vi "workbook.created_at.vi"(8 "error in":errorcluster, 11 "Workbook in":refnum<class "Workbook.lvclass">) -> (0 "error out":errorcluster, 3 "Workbook out":refnum<class "Workbook.lvclass">)   [LabVIEW 2020, in "Workbook.lvclass"]
doc: "Returns the workbook's creation time."
uses:
  Workbook.lvclass
  client.lvlib
panel:
  out "out_millis out":dbl
  in  "out_millis":dbl
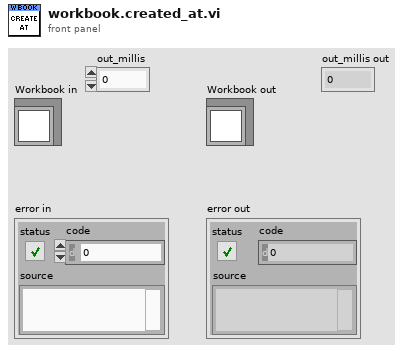
[diagram p1: front panel]
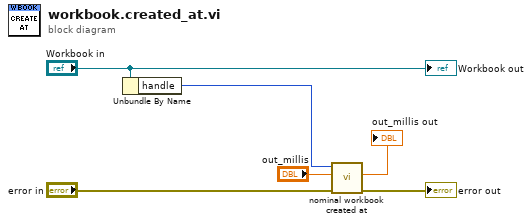
[diagram p0: block diagram]
diagram:
  n1 = Unbundle By Name("Workbook in") -> ("handle"=w4:i32)
  n2 = call "nominal workbook created at.vi"("error in (no error)"="error in", "out_millis"="out_millis", "workbook"=w4) -> ("error out"=→"error out":errorcluster, "out_millis out"=→"out_millis out":dbl)  [unwired: 6 in, 1 out]
  "Workbook out" <- "Workbook in"
